vi "NIST Time Synch (2010).vi"(4 "error in (no error)":errorcluster, 7 "Time Server IP Address (129.6.15.29)":string="129.6.15.29") -> (0 "error out":errorcluster)   [LabVIEW 2018]
uses:
  kernel32.dll
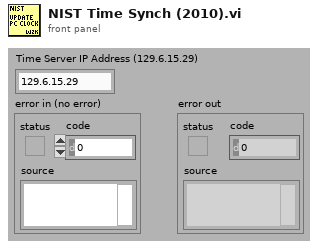
[diagram p1: front panel]
types:
  T1 = enum16{"Standard", "Buffered", "CRLF", "Immediate"}
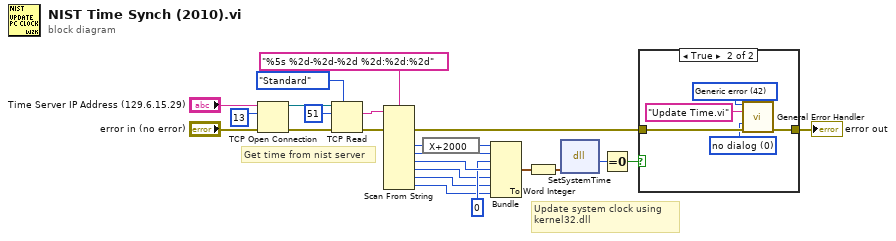
[diagram p0: block diagram]
diagram:
  # "Update system clock using \nkernel32.dll"
  # "Get time from nist server"
  n1 = TCP Open Connection(address="Time Server IP Address (129.6.15.29)", remote port or service name=u16 13 ("port"), error in (no error)="error in (no error)") -> (connection ID=w10:refnum<k5>, error out=w11:errorcluster)  [unwired: 2 in]
  n2 = TCP Read(connection ID=w10, bytes to read=51, error in (no error)=w11, 7:T1."Standard" ("mode (standard)")) -> (data out=w9:string, error out=w6:errorcluster)  [unwired: 1 in, 1 out]
  n3 = Scan From String(format string="%5s %2d-%2d-%2d %2d:%2d:%2d", input string=w9, error in=w6) -> (error out=w3:errorcluster, output 2=w23:i32, output 3=w21:i32, output 4=w20:i32, output 5=w18:i32, output 6=w17:i32, output 7=w16:i32)  [unwired: 9 in, 2 out]
  n4 = expression code="X+2000"(w23) -> (w22:i32)
  n5 = Bundle(w22, w21, 0, w20, w18, w17, w16) -> (w15:cluster{i32, i32, i32, i32, i32, i32, i32})  [unwired: 1 in]
  n6 = To Word Integer(number=w15) -> (16bit integer=w14:cluster{i16, i16, i16, i16, i16, i16, i16})
  n7 = dll-call lib="kernel32.dll" fn="SetSystemTime"("SYSTEMTIME"=w14) -> ("ERROR"=w5:i32)  [unwired: 4 in, 2 out]
  n8 = Equal To 0?(x=w5) -> (x = 0?=w2:bool)
  n9 = case shown="True" w2 {
    tunnel: w3 -> [w25 w30]
    tunnel: [w25 w29] -> w1
    frame False {
    }
    frame True {
      w27 = u16 0 items=["no dialog", "OK message", "continue or stop message"] ("type of dialog (OK msg:1)")
      w28 = 42 items=["No error", "Argument error", "Memory is full", "Out of zone", "End of file", "File already open", "Generic file I/O error", "File not found", "File permission error", "Disk is full", "Duplicate path", "Too many files open", "System feature not enabled", "Resource file not found", "Cannot add resource", "Resource not found", "Image not found", "Image memory error", "Pen does not exist", "Config type invalid", "Config token not found", "Config parse error", "Config memory error", "Bad external code format", "Bad external code offset", "External code not present", "Null window", "Destroy window error", "Null menu", "Print aborted", "Bad print record", "Print driver error", "Windows error during printing", "Memory error during printing", "Print dialog error", "Generic print error", "Invalid device refnum", "Device not found", "Device parameter error", "Device unit error", "Cannot open device", "Device call aborted", "Generic error", "Cancelled by user", "Object ID too low", "Object ID too high", "Object not in heap", "Unknown heap", "Unknown object (invalid DefProc)", "Unknown object (DefProc not in table)", "Message out of range", "Invalid (null) method", "Unknown message", "Manager call not supported", "Bad address", "Network operation in progress", "Network operation timed out", "Connection is busy", "Network attribute not supported", "Network error", "Address in use", "System out of memory", "Connection aborted", "Connection refused", "Not connected", "Already connected", "Connection closed", "Initialization error (interapplication manager)", "Bad occurrence", "Wait on unbound occurrence handler", "Occurrence queue overflow", "Datalog type conflict", "Unused", "Unrecognized type (interapplication manager)", "Memory corrupt", "Failed to make temporary DLL", "Old CIN version", "Drag socket not found", "Failed to load drop-object", "Failed to register OLE object", "Failed to release OLE object", "Format specifier type mismatch", "Unknown format specifier", "Too few format specifiers", "Too many format specifiers", "Scan failed", "Newer CIN version", "Error converting to variant", "Runtime menu error", "Password tampered", "Variant attribute not found", "Incompatible variant data type", "Event data is not available", "Event Store is not present", "Occurrence is not found", "Event Queue is not created", "Event info is not available", "Refnum passed is NULL", "Error retrieving Class GUID", "Error retrieving CoClass GUID", "Error retrieving TypeLib GUID.", "Bad built application magic bytes.", "Specific driver is different from the specific driver associated with the Logical Name.", "There is no session opened to the class driver.", "Max Error", "MAX - Error with config objects", "MAX - Error loading configuration", "MAX - Group not supported"]
      n10 = call <vilib>:"General Error Handler.vi"("[error code] (0)"=w28, "[error source] (\" \")"="Update Time.vi" ("[error source] (\" \")"), "type of dialog (OK msg:1)"=w27, "error in (no error)"=w30) -> ("error out"=w29:errorcluster)  [unwired: 7 in, 4 out]
    }
  }
  "error out" <- w1
